vi "Analog Output.vi"(1 "error in":errorcluster, 2 "output waveform":waveform(dbl)) -> ()   [LabVIEW 2024]
uses:
  <vilib>/DAQmx/write.llb/DAQmx Write (Analog Wfm 1Chan NSamp).vi
  <vilib>/DAQmx/create/channels.llb/DAQmx Create Channel (AO-Voltage-Basic).vi
  <vilib>/DAQmx/configure/timing.llb/DAQmx Timing (Sample Clock).vi
  <vilib>/DAQmx/miscellaneous.llb/DAQmx Fill In Error Info.vi
panel:
  out "number of samples written per channel":u32=1035
  in  "physical channels":tag="Dev2/ao0"
  out "Output Data":waveform(dbl)(graph)
  out "error out":errorcluster={"status"=TRUE, "code"=-200561, "source"=""}
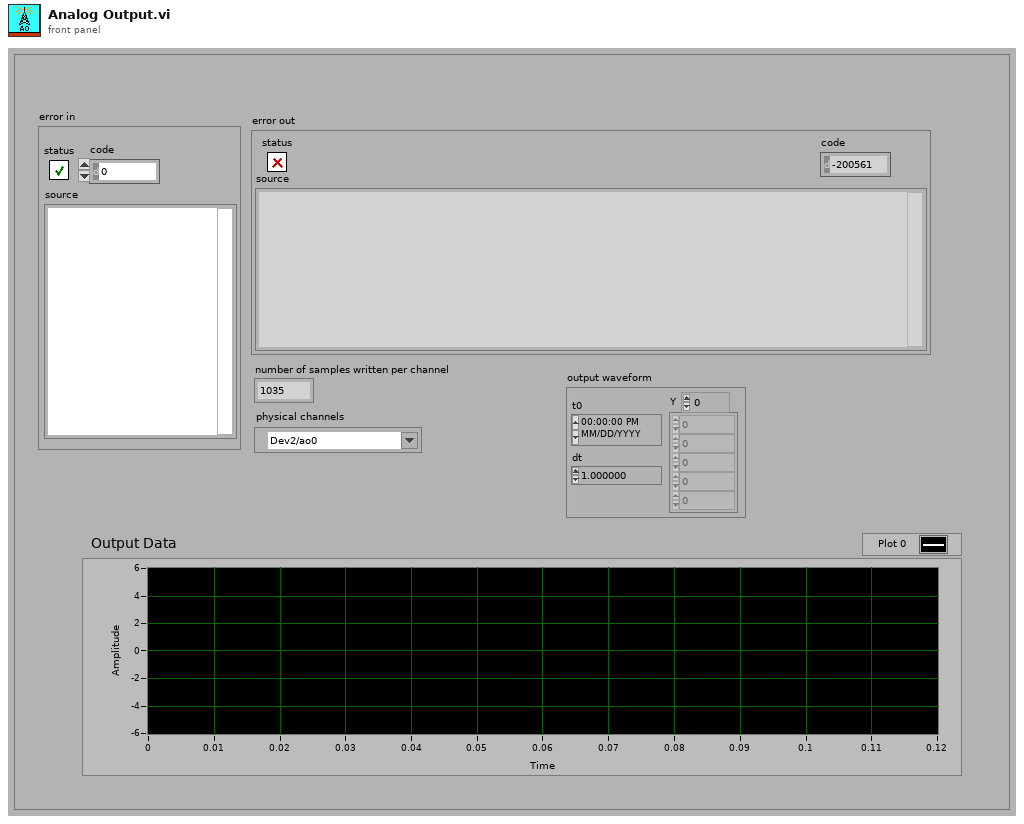
[diagram p1: front panel]
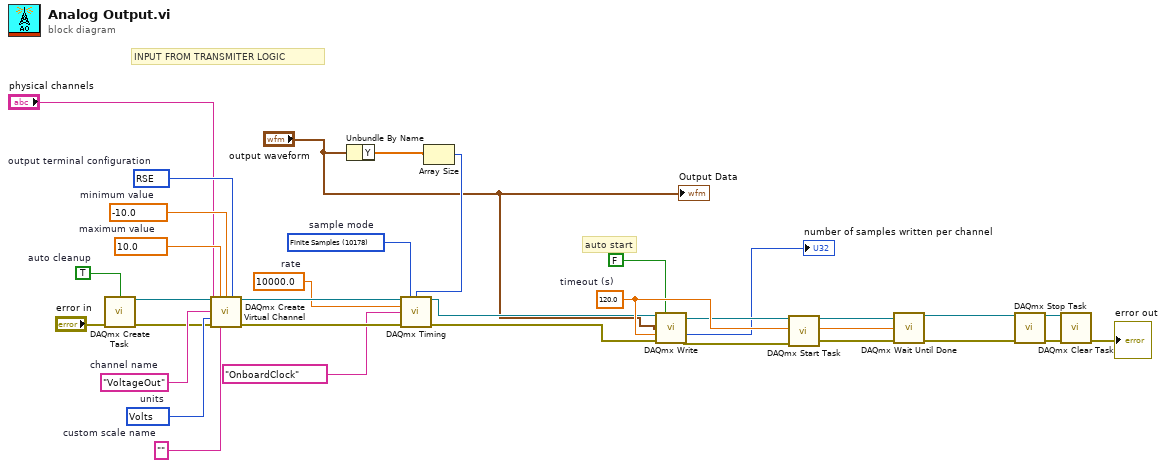
[diagram p0: block diagram]
diagram:
  w15 = 10178 items=["Finite Samples"=10178, "Continuous Samples"=10123, "Hardware Timed Single Point"=12522]  # sample mode
  w16 = 10000.0  # rate
  w25 = 10083 items=["Default"=-1, "RSE"=10083, "Differential"=10106, "Pseudodifferential"=12529]  # output terminal configuration
  w26 = 10348 items=["Volts"=10348, "From Custom Scale"=10065]  # units
  w27 = "VoltageOut"  # channel name
  w29 = ""  # custom scale name
  w30 = -10.0  # minimum value
  w31 = 10.0  # maximum value
  w32 = TRUE  # auto cleanup
  w23 = 120.0  # timeout (s)
  # "INPUT FROM TRANSMITER LOGIC"
  # "auto start"
  n1 = call <vilib>:"DAQmx Create Task.vi"("auto cleanup"=w32, "error in"="error in") -> ("task out"=w14:refnum<k21>, "error out"=w13:errorcluster)  [unwired: 12 in]
  n2 = call-poly <vilib>:"DAQmx Create Virtual Channel.vi"("task in"=w14, "maximum value"=w31, "minimum value"=w30, "output terminal configuration"=w25, "physical channels"="physical channels", "name to assign"=w27, "units"=w26, "error in"=w13, "custom scale name"=w29) -> ("task out"=w24:refnum<k21>, "error out"=w28:errorcluster)  [unwired: 5 in]
  n3 = Unbundle By Name("output waveform") -> ("Y"=w3:dbl[])
  n4 = Array Size(array=w3) -> (size(s)=w2:i32)
  n5 = call-poly <vilib>:"DAQmx Timing.vi"("task/channels in"=w24, "sample mode"=w15, "samples per channel"=w2, "rate"=w16, "source"=tag "OnboardClock", "error in"=w28) -> ("task out"=w7:refnum<k21>, "error out"=w6:errorcluster)  [unwired: 8 in]
  n6 = call-poly <vilib>:"DAQmx Write.vi"("task/channels in"=w7, "auto start"=FALSE, "data"="output waveform", "timeout"=w23, "error in"=w6) -> ("task out"=w9:refnum<k21>, "number of samples written per channel"=→"number of samples written per channel":u32, "error out"=w8:errorcluster)  [unwired: 8 in]
  n7 = call <vilib>:"DAQmx Start Task.vi"("task/channels in"=w9, "error in"=w8) -> ("task out"=w10:refnum<k21>, "error out"=w11:errorcluster)  [unwired: 12 in]
  n8 = call <vilib>:"DAQmx Wait Until Done.vi"("task/channels in"=w10, "timeout (sec)"=w23, "error in"=w11) -> ("task out"=w22:refnum<k21>, "error out"=w21:errorcluster)  [unwired: 11 in]
  n9 = call <vilib>:"DAQmx Stop Task.vi"("task/channels in"=w22, "error in"=w21) -> ("task out"=w18:refnum<k21>, "error out"=w19:errorcluster)  [unwired: 12 in]
  n10 = call <vilib>:"DAQmx Clear Task.vi"("task in"=w18, "error in"=w19) -> ("error out"=→"error out":errorcluster)  [unwired: 13 in]
  "Output Data" <- "output waveform"
